vi "Calc Pitch.vi"(10 "Position":dbl) -> (2 "Pitch":dbl)   [LabVIEW 2014]
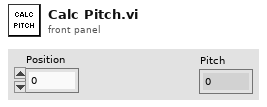
[diagram p1: front panel]
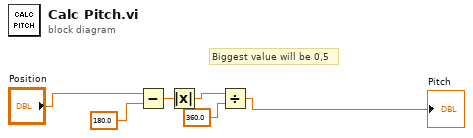
[diagram p0: block diagram]
diagram:
  # "Biggest value will be 0,5"
  n1 = Subtract(x="Position", y=180.0) -> (x-y=w4:dbl)
  n2 = Absolute Value(x=w4) -> (abs(x)=w3:dbl)
  n3 = Divide(x=w3, y=360.0) -> (x/y=→"Pitch":dbl)
